vi "InitializeSubpanels.vi"(8 "error in (no error)":errorcluster, 11 "Maui Manager in":refnum<class "Maui Manager.lvclass">) -> (0 "error out":errorcluster, 3 "Maui Manager out":refnum<class "Maui Manager.lvclass">)   [LabVIEW 2020, in "Maui Manager.lvclass"]
uses:
  Maui Manager.lvclass
  Maui Manager.lvclass/Maui Manager.ctl
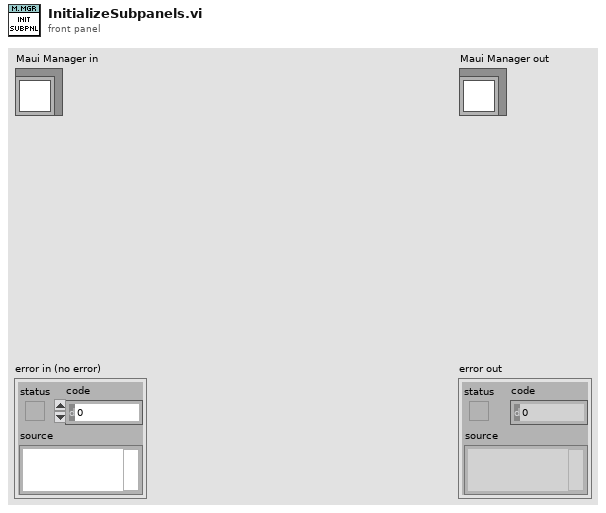
[diagram p1: front panel]
types:
  T1 = cluster{"Control":refnum<vi>, "Subpanel":refnum<vi>, "Active":i32, "Ctrl Class":string}[]
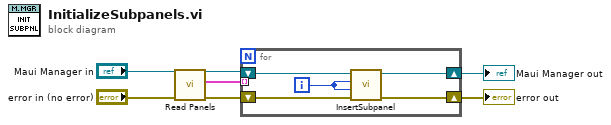
[diagram p0: block diagram]
diagram:
  n1 = call "Read Panels.vi"("error in (no error)"="error in (no error)", "Maui Manager in"="Maui Manager in") -> ("error out"=w4:errorcluster, "Panels"=w3:T1, "Maui Manager out"=w6:refnum<class "Maui Manager.lvclass">)  [unwired: 7 in]
  n2 = for {
    shift-right: [w11] -> w2
    shift-left: w6 -> [w12]
    shift-right: [w9] -> w1
    shift-left: w4 -> [w10]
    tunnel: w3 -> [_] mode=indexing
    i -> [w8]
    n3 = call "InsertSubpanel.vi"("error in (no error)"=w10, "Subpanel"=w8, "Panel"=w8, "Maui Manager in"=w12) -> ("error out"=w9:errorcluster, "Maui Manager out"=w11:refnum<class "Maui Manager.lvclass">)  [unwired: 6 in]
  }
  "error out" <- w1
  "Maui Manager out" <- w2
